vi "电流加载及换向回读.vi"(0 "6510 in":refnum<visa-resource-name>, 1 "TDK in":refnum<visa-resource-name>, 2 "输入电流":dbl, 3 "Delay Time (s)":dbl=1.0 caption="延迟时间(s)", 4 "电源台数":u8=1, 5 "error in":errorcluster, 6 "modbusin":refnum<visa-resource-name>="COM5", 7 "y":dbl=5000.0 format="%#_13g") -> (14 "2700 out":refnum<visa-resource-name>, 15 "TDK out":refnum<visa-resource-name>, 16 "实际电流":dbl, 19 "error out":errorcluster)   [LabVIEW 2021]
uses:
  <vilib>/NI/Modbus Library/API/Wrapper/Create Serial Master.vi
  <instrlib>/Keithley 27XX/Public/Data/Read Single Point.vi
  <vilib>/NI/Modbus Library/API/Master/Modbus Master.lvclass
  <vilib>/NI/Modbus Library/API/Wrapper/API Main.lvlib
  <instrlib>/TDK-Lambda G Series/TDK-Lambda G Series.lvlib
  <instrlib>/Keithley 27XX/Keithley 27XX.lvlib
panel:
  out "x*y":dbl
  # "TDK 电流加载及换向"
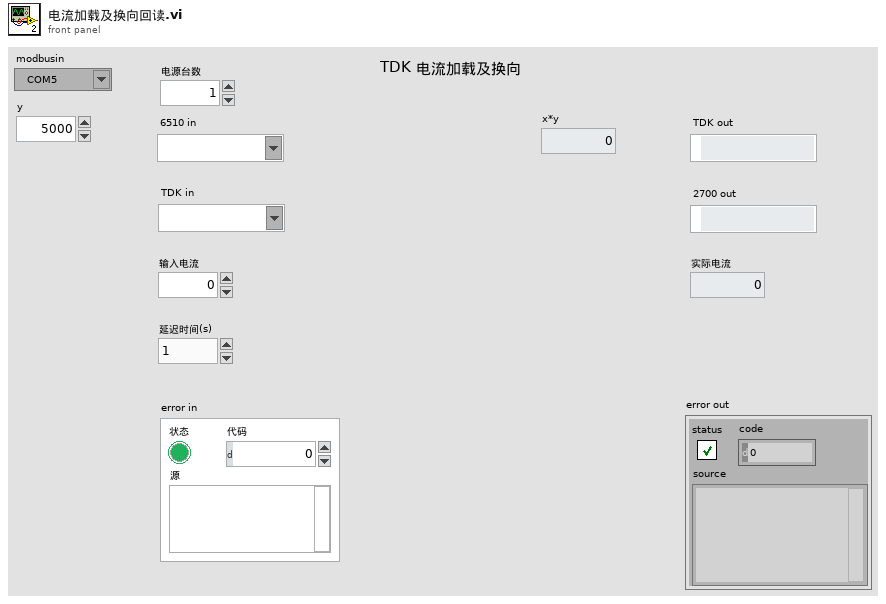
[diagram p1: front panel]
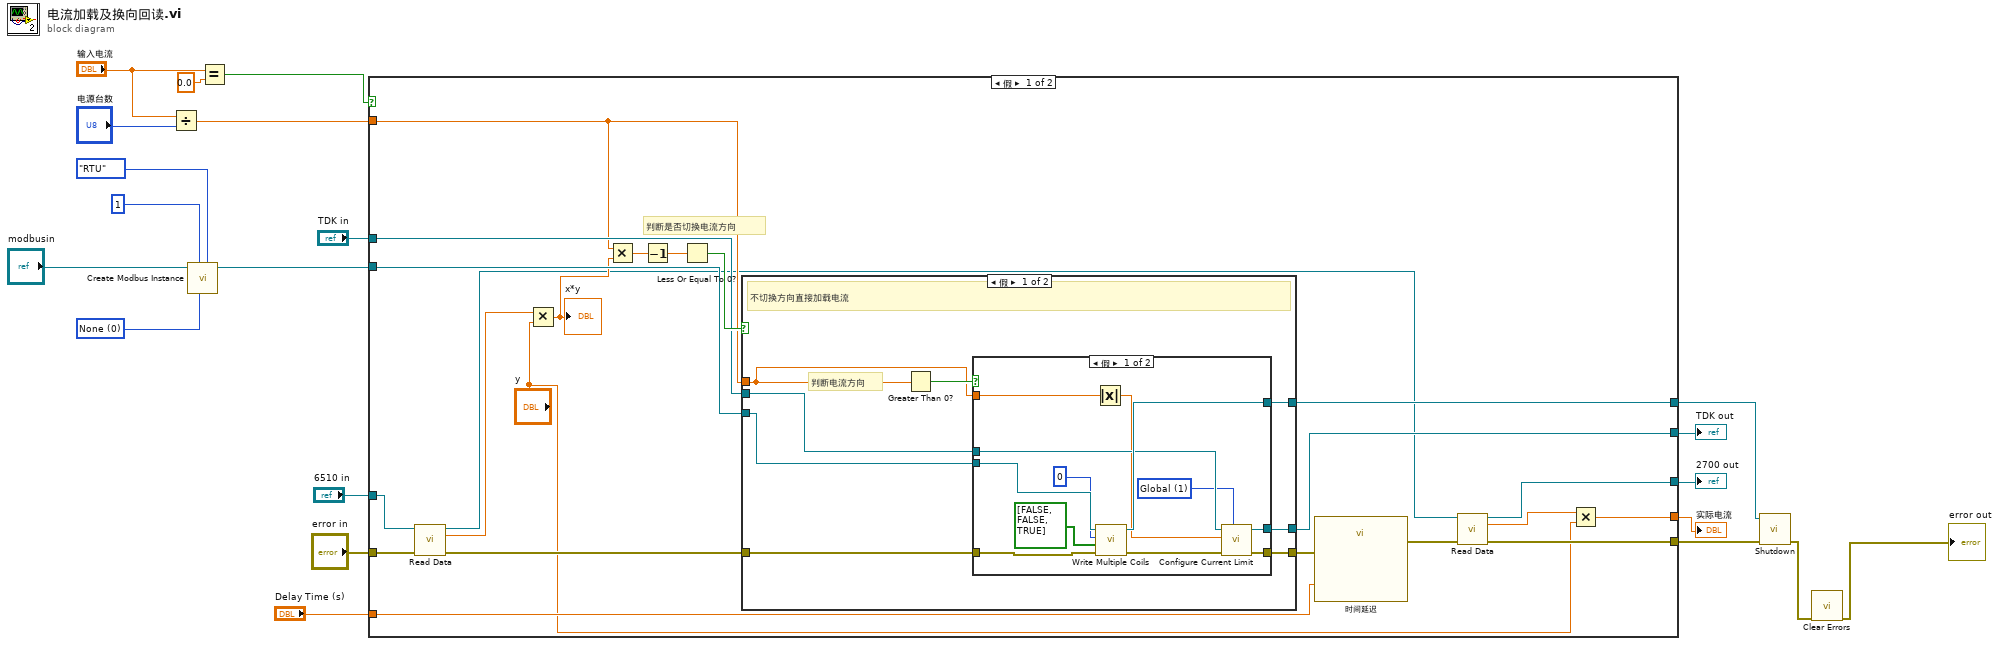
[diagram p0: block diagram]
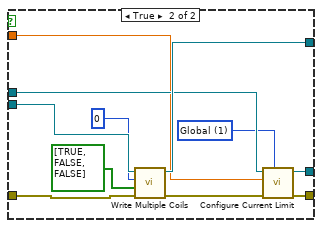
[diagram p2: hidden frame]
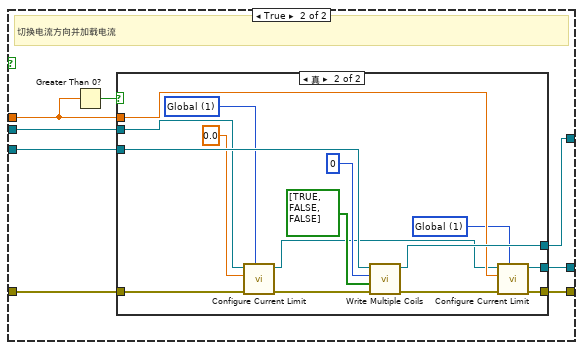
[diagram p3: hidden frame]
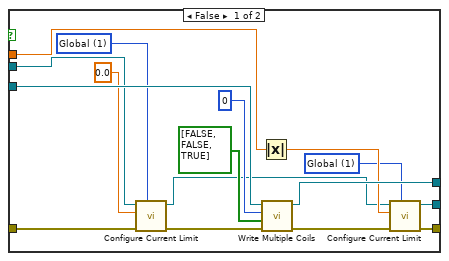
[diagram p4: hidden frame]
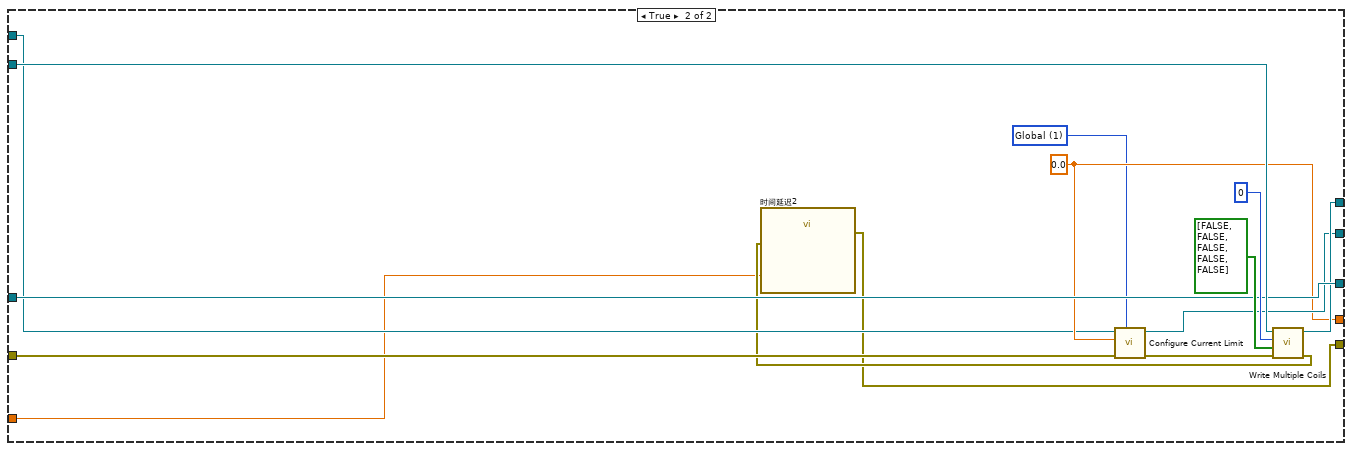
[diagram p5: hidden frame]
diagram:
  w11 = u16 0 items=["None", "Odd", "Even", "Mark", "Space"] ("parity (even)")
  n1 = Divide(x="输入电流", y="电源台数") -> (x/y=w3:dbl)
  n2 = call-poly <vilib>:"Create Modbus Instance.vi"("serial type"=enum16{"RTU", "ASCII"}."RTU", "parity (even)"=w11, "unit ID"=u8 1, "VISA resource name"="modbusin") -> ("serial master instance"=w15:refnum<class "Modbus Master.lvclass">)  [unwired: 6 in, 1 out]
  n3 = Equal?(x="输入电流", y=0.0) -> (x = y?=w17:bool)
  n4 = case shown="假" w17 {
    tunnel: "TDK in" -> [w40 w118]
    tunnel: w15 -> [w39 w127]
    tunnel: [w25 w115] -> w7
    tunnel: "Delay Time (s)" -> [w37 w114]
    tunnel: "error in" -> [w29 w121]
    tunnel: [w36 w122] -> w19
    tunnel: "6510 in" -> [w30 w124]
    tunnel: [w24 w124] -> w10
    tunnel: w3 -> [w35 _]
    tunnel: [w32 w119] -> w16
    tunnel: [w34 w123] -> w9
    frame False {
      # "判断是否切换电流方向"
      n5 = call-poly <instrlib>:"Read Data.vi"("VISA resource name"=w30, "error in (no error)"=w29) -> ("VISA resource name out"=w27:refnum<visa-resource-name>, "Measurement Data"=w31:dbl, "error out"=w28:errorcluster)  [unwired: 11 in]
      n6 = Multiply(x=w31, y="y") -> (x*y=w33:dbl)
      "x*y" <- w33
      n7 = Multiply(x=w35, y=w33) -> (x*y=w42:dbl)
      n8 = Decrement(x=w42) -> (x-1=w41:dbl)
      n9 = Less Or Equal To 0?(x=w41) -> (x <= 0?=w43:bool)
      n10 = case shown="假" w43 {
        tunnel: w35 -> [w50 w82]
        tunnel: w28 -> [w47 w77]
        tunnel: w40 -> [w49 w80]
        tunnel: w39 -> [w45 w79]
        tunnel: [w48 w78] -> w38
        tunnel: [w46 w76] -> w36
        tunnel: [w44 w75] -> w34
        frame False {
          # "判断电流方向"
          # "不切换方向直接加载电流"
          n11 = Greater Than 0?(x=w50) -> (x > 0?=w51:bool)
          n12 = case shown="假" w51 {
            tunnel: w50 -> [w63 w67]
            tunnel: w49 -> [w56 w68]
            tunnel: [w53 w65] -> w48
            tunnel: w47 -> [w58 w73]
            tunnel: [w57 w69] -> w46
            tunnel: w45 -> [w62 w74]
            tunnel: [w61 w70] -> w44
            frame False {
              w52 = u16 1 items=["Single", "Global"] ("Globalize (0: Single)")
              n13 = Absolute Value(x=w63) -> (abs(x)=w55:dbl)
              n14 = call-dynamic "Write Multiple Coils.vi"("error in"=w58, "coils to write"=bool[] [FALSE, FALSE, TRUE], "starting address"=u16 0, "Modbus master in"=w62) -> ("error out"=w54:errorcluster, "Modbus master out"=w61:refnum<class "Modbus Master.lvclass">)  [unwired: 6 in]
              n15 = call <instrlib>:"Configure Current Limit.vi"("Globalize (0: Single)"=w52, "error in (no error)"=w54, "Current Limit (0A)"=w55, "VISA resource name"=w56) -> ("error out"=w53:errorcluster, "VISA resource name out"=w57:refnum<visa-resource-name>)  [unwired: 6 in]
            }
            frame True {
              w64 = u16 1 items=["Single", "Global"] ("Globalize (0: Single)")
              n16 = call-dynamic "Write Multiple Coils.vi"("error in"=w73, "coils to write"=bool[] [TRUE, FALSE, FALSE], "starting address"=u16 0, "Modbus master in"=w74) -> ("error out"=w66:errorcluster, "Modbus master out"=w70:refnum<class "Modbus Master.lvclass">)  [unwired: 6 in]
              n17 = call <instrlib>:"Configure Current Limit.vi"("Globalize (0: Single)"=w64, "error in (no error)"=w66, "Current Limit (0A)"=w67, "VISA resource name"=w68) -> ("error out"=w65:errorcluster, "VISA resource name out"=w69:refnum<visa-resource-name>)  [unwired: 6 in]
            }
          }
        }
        frame True {
          # "切换电流方向并加载电流"
          n18 = Greater Than 0?(x=w82) -> (x > 0?=w81:bool)
          n19 = case shown="真" w81 {
            tunnel: w82 -> [w97 w107]
            tunnel: w80 -> [w87 w105]
            tunnel: w79 -> [w96 w111]
            tunnel: [w93 w109] -> w78
            tunnel: w77 -> [w85 w103]
            tunnel: [w92 w108] -> w76
            tunnel: [w95 w110] -> w75
            frame False {
              w83 = u16 1 items=["Single", "Global"] ("Globalize (0: Single)")
              w84 = u16 1 items=["Single", "Global"] ("Globalize (0: Single)")
              n20 = call <instrlib>:"Configure Current Limit.vi"("Globalize (0: Single)"=w83, "error in (no error)"=w85, "Current Limit (0A)"=0.0 ("Curr(0)"), "VISA resource name"=w87) -> ("error out"=w89:errorcluster, "VISA resource name out"=w88:refnum<visa-resource-name>)  [unwired: 6 in]
              n21 = Absolute Value(x=w97) -> (abs(x)=w91:dbl)
              n22 = call-dynamic "Write Multiple Coils.vi"("error in"=w89, "coils to write"=bool[] [FALSE, FALSE, TRUE] ("coil values"), "starting address"=u16 0, "Modbus master in"=w96) -> ("error out"=w90:errorcluster, "Modbus master out"=w95:refnum<class "Modbus Master.lvclass">)  [unwired: 6 in]
              n23 = call <instrlib>:"Configure Current Limit.vi"("Globalize (0: Single)"=w84, "error in (no error)"=w90, "Current Limit (0A)"=w91, "VISA resource name"=w88) -> ("error out"=w93:errorcluster, "VISA resource name out"=w92:refnum<visa-resource-name>)  [unwired: 6 in]
            }
            frame True {
              w99 = u16 1 items=["Single", "Global"] ("Globalize (0: Single)")
              w100 = u16 1 items=["Single", "Global"] ("Globalize (0: Single)")
              n24 = call <instrlib>:"Configure Current Limit.vi"("Globalize (0: Single)"=w99, "error in (no error)"=w103, "Current Limit (0A)"=0.0 ("Curr(0)"), "VISA resource name"=w105) -> ("error out"=w102:errorcluster, "VISA resource name out"=w101:refnum<visa-resource-name>)  [unwired: 6 in]
              n25 = call-dynamic "Write Multiple Coils.vi"("error in"=w102, "coils to write"=bool[] [TRUE, FALSE, FALSE] ("coil values"), "starting address"=u16 0, "Modbus master in"=w111) -> ("error out"=w106:errorcluster, "Modbus master out"=w110:refnum<class "Modbus Master.lvclass">)  [unwired: 6 in]
              n26 = call <instrlib>:"Configure Current Limit.vi"("Globalize (0: Single)"=w100, "error in (no error)"=w106, "Current Limit (0A)"=w107, "VISA resource name"=w101) -> ("error out"=w109:errorcluster, "VISA resource name out"=w108:refnum<visa-resource-name>)  [unwired: 6 in]
            }
          }
        }
      }
      n27 = call "时间延迟"("error in (no error)"=w38, "Delay Time (s)"=w37) -> ("error out"=w26:errorcluster)  [unwired: 9 in]
      n28 = call-poly <instrlib>:"Read Data.vi"("VISA resource name"=w27, "error in (no error)"=w26) -> ("VISA resource name out"=w24:refnum<visa-resource-name>, "Measurement Data"=w23:dbl, "error out"=w25:errorcluster)  [unwired: 11 in]
      n29 = Multiply(x=w23, y="y") -> (x*y=w32:dbl)
    }
    frame True {
      w117 = u16 1 items=["Single", "Global"] ("Globalize (0: Single)")
      w119 = 0.0 ("Curr(0)")
      n30 = call <instrlib>:"Configure Current Limit.vi"("Globalize (0: Single)"=w117, "error in (no error)"=w121, "Current Limit (0A)"=w119, "VISA resource name"=w118) -> ("error out"=w120:errorcluster, "VISA resource name out"=w122:refnum<visa-resource-name>)  [unwired: 6 in]
      n31 = call-dynamic "Write Multiple Coils.vi"("error in"=w120, "coils to write"=bool[] [FALSE, FALSE, FALSE, FALSE, FALSE] ("coil values"), "starting address"=u16 0, "Modbus master in"=w127) -> ("error out"=w116:errorcluster, "Modbus master out"=w123:refnum<class "Modbus Master.lvclass">)  [unwired: 6 in]
      n32 = call "时间延迟2"("error in (no error)"=w116, "Delay Time (s)"=w114) -> ("error out"=w115:errorcluster)  [unwired: 9 in]
    }
  }
  "实际电流" <- w16
  "TDK out" <- w19
  "2700 out" <- w10
  n33 = call-dynamic "Shutdown.vi"("error in"=w7, "Modbus master in"=w9) -> ("error out"=w2:errorcluster)  [unwired: 9 in]
  n34 = call <vilib>:"Clear Errors.vi"("error in (no error)"=w2) -> ("error out"=→"error out":errorcluster)  [unwired: 5 in, 1 out]
